vi "iWorx Pulse SubVI.vi"(5 "Waveform Array Chart":refnum<vi>, 7 "Selection Chart":refnum<vi>, 10 "Threshold (.5mV)":dbl=0.0005) -> (1 "Pulse Times":timestamp[](array[timestamp]), 2 "Inst Pulse Rate (BPM)":dbl, 3 "Average Pulse Rate (BPM)":dbl)   [LabVIEW 2012]
doc: "This subVI uses a Reference from a Waveform Chart in order to extract the data visible on the chart. It then calculates when pulse beats occur based on a simple negative threshold. This function returns the <b>Instantaneous Pulse</b> based on your last two heart beats as well as the <b>Average Pulse</b> from the data visible on the chart."
panel:
  out "Error Out":errorcluster
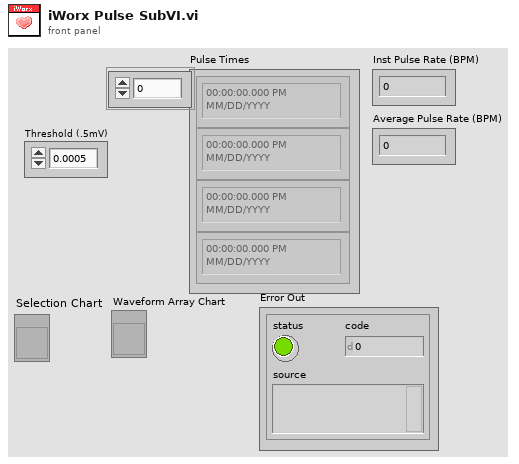
[diagram p1: front panel]
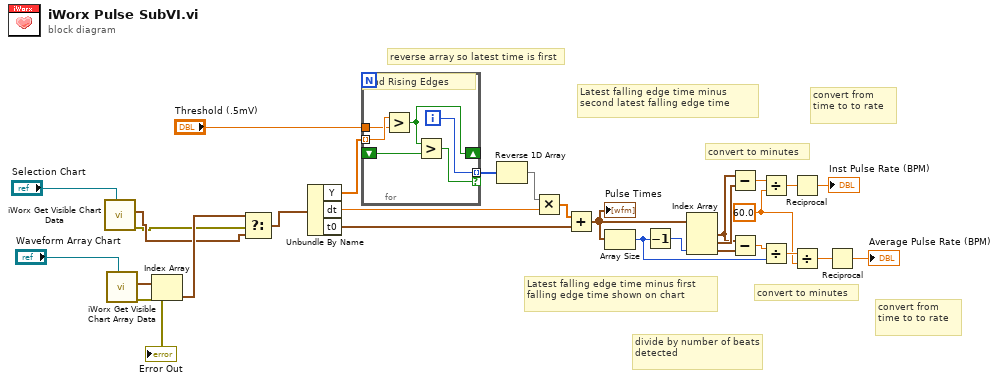
[diagram p0: block diagram]
diagram:
  w15 = 60.0 ("y")
  # "reverse array so latest time is first"
  # "convert to minutes"
  # "divide by number of beats detected"
  # "convert from time to to rate"
  # "convert from time to to rate"
  # "convert to minutes"
  # "Latest falling edge time minus first falling edge time shown on chart"
  # "Latest falling edge time minus second latest falling edge time"
  n1 = call "iWorx Get Visible Chart Data.vi"("Selection Chart"="Selection Chart") -> ("Error Out"=w2:errorcluster, "Waveform out"=w4:waveform(dbl))  [unwired: 8 in, 1 out]
  n2 = call "iWorx Get Visible Chart Array Data.vi"("Waveform Chart 3"="Waveform Array Chart") -> ("Error Out"=→"Error Out":errorcluster, "Waveforms Out"=w6:waveform(dbl)[])  [unwired: 9 in]
  n3 = Index Array(array=w6) -> (element=w5:waveform(dbl))  [unwired: 1 in]
  n4 = Select(t=w5, s=w2, f=w4) -> (s? t:f=w3:waveform(dbl))
  n5 = Unbundle By Name(w3) -> ("Y"=w29:dbl[], "dt"=w28:dbl, "t0"=w26:timestamp)
  n6 = for {
    tunnel: w29 -> [w35] mode=indexing
    tunnel: "Threshold (.5mV)" -> [w34]
    shift-right: [w33] -> _
    shift-left: _ -> [w32]
    tunnel: [w31] -> w25 mode=indexing if=w30
    i -> [w31]
    # "Find Rising Edges"
    n7 = Greater?(x=w35, y=w34) -> (0:w33:bool)
    n8 = Greater?(x=w33, y=w32) -> (0:w30:bool)
  }
  n9 = Reverse 1D Array(array=w25) -> (reversed array=w24:i32[])
  n10 = Multiply(x=w24, y=w28) -> (x*y=w27:dbl[])
  n11 = Add(x=w27, y=w26) -> (x+y=w12:timestamp[])
  "Pulse Times" <- w12
  n12 = Array Size(array=w12) -> (size(s)=w17:i32)
  n13 = Decrement(x=w17) -> (x-1=w23:i32)
  n14 = Index Array(array=w12, index #3=w23) -> (element #1=w21:timestamp, element #2=w22:timestamp, element #3=w20:timestamp)  [unwired: 2 in]
  n15 = Subtract(x=w21, y=w22) -> (x-y=w19:dbl)
  n16 = Subtract(x=w21, y=w20) -> (x-y=w18:dbl)
  n17 = Divide(x=w19, y=w15) -> (x/y=w14:dbl)
  n18 = Divide(x=w18, y=w17) -> (x/y=w16:dbl)
  n19 = Reciprocal(x=w14) -> (1/x=→"Inst Pulse Rate (BPM)":dbl)
  n20 = Divide(x=w16, y=w15) -> (x/y=w13:dbl)
  n21 = Reciprocal(x=w13) -> (1/x=→"Average Pulse Rate (BPM)":dbl)
